vi "Transmission(Theta) (SubVI).vi"(3 "Theta":dbl, 8 "ParameterA":dbl=0.9936979745747752, 10 "ParameterB":dbl=1.159030509225965e-24, 12 "ParameterC":dbl=2.739352344405108, 14 "ParameterPhi":dbl=75.96290439475945) -> (23 "Transmission":dbl=1.0)   [LabVIEW 2017]
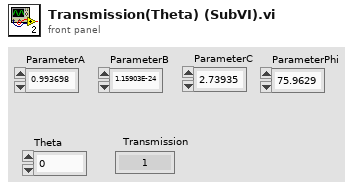
[diagram p1: front panel]
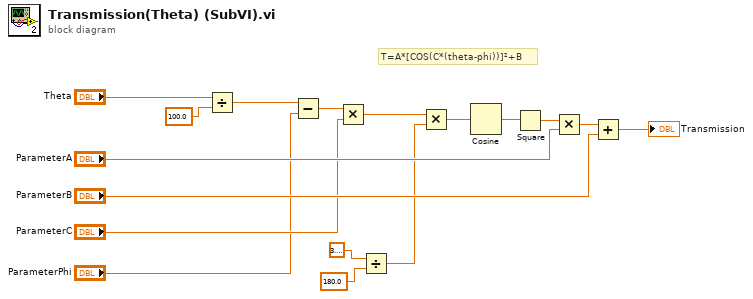
[diagram p0: block diagram]
diagram:
  # "T=A*[COS(C*(theta-phi))]²+B"
  n1 = Divide(x="Theta", y=100.0) -> (x/y=w5:dbl)
  n2 = Subtract(x=w5, y="ParameterPhi") -> (x-y=w10:dbl)
  n3 = Multiply(x=w10, y="ParameterC") -> (x*y=w7:dbl)
  n4 = Divide(x=3.141592653589793, y=180.0) -> (x/y=w6:dbl)
  n5 = Multiply(x=w7, y=w6) -> (x*y=w8:dbl)
  n6 = Cosine(x=w8) -> (cos(x)=w12:dbl)
  n7 = Square(x=w12) -> (x^2=w13:dbl)
  n8 = Multiply(x=w13, y="ParameterA") -> (x*y=w15:dbl)
  n9 = Add(x=w15, y="ParameterB") -> (x+y=→"Transmission":dbl)
